vi "InitializeDoor.vi"(8 "error in (no error)":errorcluster, 9 "r1":refnum<data-value>, 10 "r2":refnum<data-value>, 11 "Door in":refnum<class "Door.lvclass">) -> (0 "error out":errorcluster, 3 "Door out":refnum<class "Door.lvclass">)   [LabVIEW 2016, in "Door.lvclass"]
uses:
  Door.lvclass
  Room/Room.lvclass
  Door.lvclass/Door.ctl
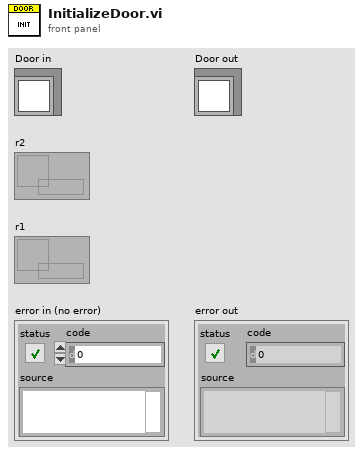
[diagram p1: front panel]
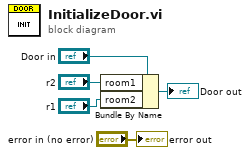
[diagram p0: block diagram]
diagram:
  n1 = Bundle By Name(cluster="Door in", "room1"="r2", "room2"="r1") -> (→"Door out":refnum<class "Door.lvclass">)
  "error out" <- "error in (no error)"
